vi "central core - noise.vi"() -> ()   [LabVIEW 2020]
uses:
  <vilib>/Analysis/3filter.llb/Filter Passband Type.ctl
  <vilib>/Utility/miscctls.llb/LVPointDoubleTypeDef.ctl
  <vilib>/Analysis/3filter.llb/Butterworth Filter (DBL).vi
  <vilib>/express/express analysis/Spectral/Block/exnSpectralBlock spectral measurements peak poly.vi
  <vilib>/express/express analysis/Spectral/Block/exnSpectralBlock spectral measurements peak WFM.vi
  <vilib>/express/express analysis/Spectral/XNode/ExpressSpectralMeasurementsBlockNode.xnode
  <vilib>/Analysis/NI_AALBase.lvlib
panel:
  out "Intensity Graph 3":dbl[][](graph)
  out "min value 2":dbl
  out "max value 2":dbl
  in  "low cutoff freq: fl":dbl=0.04 format="%#_13g"
  in  "order":i32=2
  in  "Array 3":cluster{dbl, "Color Box":u32}[](array[cluster])=[{1000.0, "Color Box"=16714752}, {750.0, "Color Box"=15859456}, {500.0, "Color Box"=65289}, {250.0, "Color Box"=983260}, {0.0, "Color Box"=14418124}]
  out "min value":dbl
  out "max value":dbl
  out "Array 2":dbl[][](array[numeric])
  out "Intensity Graph 2":dbl[][](graph)
  out "Waveform Graph 2":cluster{"f0":dbl, "df":dbl, "magnitude":dbl[]}(graph)
  out "Waveform Graph":cluster{"f0":dbl, "df":dbl, "magnitude":dbl[]}(graph)
  in  "Array":cluster{dbl, "Color Box":u32}[](array[cluster])=[{1000.0, "Color Box"=16714752}, {750.0, "Color Box"=15859456}, {500.0, "Color Box"=65289}, {250.0, "Color Box"=983260}, {0.0, "Color Box"=14418124}]
  out "output array":i16[](array[numeric])
  out "Image Pixels (I16) 2":i16[][](array[numeric])=[[45, 30, 48, 80, 127, 195, 237, 243, 154, 70, 122, 104, 194, 367, 352, 240, 149, 87, 63, 47, 92, 128, 128, 67, 39, 52, 45, 67, 104, 115], [50, 50, 64, 99, 81, 152, 118, 120, 92, 116, 64, 71, 100, 191, 192, 242, 150, 97, 76, 40, 47, 55, 45, 39, 54, 45, 64, 99, 149, 224], [37, 41, 43, 52, 61, 157, 144, 370, 413, 328, 136, 74, 77, 132, 154, 226, 274, 264, 263, 93, 47, 39, 36, 41, 45, 54, 64, 181, 262, 261], [57, 33, 48, 57, 36, 126, 400, 1139, 1471, 990, 426, 117, 68, 53, 213, 482, 730, 682, 502, 228, 70, 43, 50, 38, 46, 45, 63, 164, 233, 323], [42, 47, 36, 38, 50, 178, 708, 1307, 1980, 1298, 498, 186, 54, 79, 129, 508, 738, 836, 511, 332, 56, 51, 33, 48, 46, 47, 66, 133, 218, 251], [43, 33, 45, 58, 55, 122, 556, 966, 1092, 996, 478, 113, 88, 151, 232, 492, 730, 765, 572, 222, 84, 78, 52, 30, 29, 62, 43, 68, 94, 139], [49, 52, 36, 36, 42, 54, 167, 450, 516, 342, 265, 188, 394, 658, 854, 1048, 1097, 1085, 832, 485, 363, 136, 70, 48, 40, 27, 38, 48, 79, 82], [60, 41, 42, 40, 46, 44, 41, 105, 182, 261, 357, 707, 1036, 1348, 1662, 1687, 1948, 1605, 1319, 1576, 1082, 834, 344, 134, 50, 36, 42, 42, 48, 46], [36, 44, 51, 30, 51, 50, 58, 83, 234, 508, 950, 1428, 1764, 2324, 2186, 2166, 1882, 2127, 2020, 2238, 1880, 1490, 821, 427, 175, 65, 46, 45, 55, 56], [37, 42, 32, 33, 51, 44, 57, 161, 462, 1128, 1498, 1986, 2464, 2893, 2630, 2418, 2646, 3225, 3069, 2846, 2336, 1746, 1504, 1070, 494, 145, 72, 63, 36, 43], [50, 37, 40, 43, 41, 58, 120, 420, 986, 1616, 2419, 2510, 2533, 2588, 2872, 3422, 3455, 3263, 3008, 2527, 2411, 2560, 2122, 1861, 1150, 286, 77, 53, 41, 53], [40, 55, 58, 58, 46, 83, 257, 714, 1634, 1980, 2313, 2530, 2628, 2636, 3318, 3418, 3324, 3034, 2596, 2848, 2808, 3001, 2491, 1980, 1384, 651, 237, 40, 34, 48], [44, 40, 44, 45, 50, 130, 486, 1128, 1949, 2100, 2610, 2510, 3384, 3673, 3467, 3123, 2938, 2866, 3213, 3121, 3392, 3152, 2452, 1939, 1721, 1198, 510, 79, 41, 48], [33, 41, 40, 49, 45, 192, 763, 1254, 2019, 2332, 3095, 3363, 3632, 3650, 3081, 2909, 2967, 3495, 3610, 3411, 3053, 2633, 2652, 2554, 2042, 1442, 466, 78, 47, 45], [40, 46, 38, 43, 53, 203, 765, 1322, 1856, 2833, 3374, 3241, 3166, 2623, 2860, 3043, 3433, 3752, 3424, 2841, 2804, 2808, 3333, 2706, 2266, 1405, 691, 209, 52, 56], [42, 35, 46, 48, 75, 238, 777, 1499, 2356, 3159, 3058, 3150, 2850, 2866, 3378, 3538, 3456, 2992, 2823, 3076, 2986, 3476, 3549, 2923, 2054, 1364, 838, 259, 56, 70], [36, 46, 37, 48, 69, 183, 1109, 1898, 2624, 3005, 3002, 2850, 3306, 3476, 3378, 3509, 3199, 2884, 3449, 3510, 3308, 3642, 3143, 2620, 2131, 1809, 860, 256, 47, 56], [42, 44, 43, 38, 84, 216, 821, 1625, 2029, 2406, 2878, 3224, 3503, 3374, 3210, 2938, 2980, 3197, 3439, 3390, 3404, 3034, 2714, 2623, 2344, 1635, 1008, 185, 48, 47], [40, 67, 59, 58, 48, 210, 704, 1509, 1735, 2306, 3292, 3575, 3479, 3134, 2673, 3230, 3674, 3662, 3280, 3200, 2832, 3156, 3285, 2921, 2536, 1602, 722, 182, 49, 51], [46, 142, 147, 151, 72, 138, 433, 1157, 1793, 2633, 3124, 2894, 2851, 2854, 3294, 3636, 3774, 3640, 2965, 3071, 3170, 3313, 3315, 2559, 1880, 1187, 624, 85, 70, 43], [124, 201, 271, 363, 90, 64, 313, 820, 1802, 2216, 2614, 2334, 2950, 3845, 3980, 3365, 3359, 3001, 2949, 3217, 3262, 3548, 2841, 1976, 1393, 866, 296, 48, 47, 52], [132, 260, 538, 366, 212, 52, 135, 503, 1232, 1586, 2206, 2650, 3290, 3425, 3241, 2896, 2798, 3116, 3736, 3408, 3253, 2753, 2403, 1853, 1067, 564, 192, 58, 57, 35], [125, 225, 463, 371, 191, 78, 59, 238, 521, 1406, 1790, 2423, 2876, 2804, 2840, 3005, 3432, 3702, 3552, 3440, 2800, 2220, 1832, 1311, 826, 289, 82, 69, 44, 45], [99, 206, 331, 285, 222, 128, 264, 351, 516, 764, 1412, 2020, 2044, 2224, 2589, 2906, 2986, 3320, 2702, 2370, 2126, 1960, 1561, 672, 281, 75, 56, 38, 42, 47], [50, 64, 148, 147, 104, 132, 417, 735, 510, 468, 668, 893, 1382, 1918, 2400, 2465, 2452, 2236, 2205, 1993, 1615, 1078, 648, 239, 96, 49, 47, 36, 41, 50], [48, 56, 43, 67, 60, 150, 351, 731, 616, 378, 186, 384, 752, 878, 1230, 1220, 1315, 1364, 1133, 1140, 840, 448, 162, 66, 40, 36, 57, 50, 40, 43], [53, 47, 48, 59, 32, 90, 196, 410, 484, 183, 91, 60, 212, 250, 340, 452, 628, 495, 450, 302, 173, 86, 63, 43, 45, 43, 40, 41, 40, 42], [38, 38, 42, 37, 44, 46, 78, 142, 149, 115, 70, 52, 59, 54, 66, 80, 97, 69, 72, 46, 59, 50, 44, 55, 51, 40, 34, 42, 45, 39], [47, 42, 37, 50, 50, 42, 59, 53, 81, 41, 36, 52, 44, 62, 53, 44, 40, 42, 42, 47, 38, 47, 38, 55, 39, 57, 48, 41, 45, 47], [48, 47, 40, 37, 40, 50, 42, 35, 38, 48, 37, 61, 42, 53, 31, 46, 35, 38, 45, 37, 38, 34, 40, 32, 50, 36, 40, 57, 42, 46]]
  out "Intensity Graph":i16[][](graph)
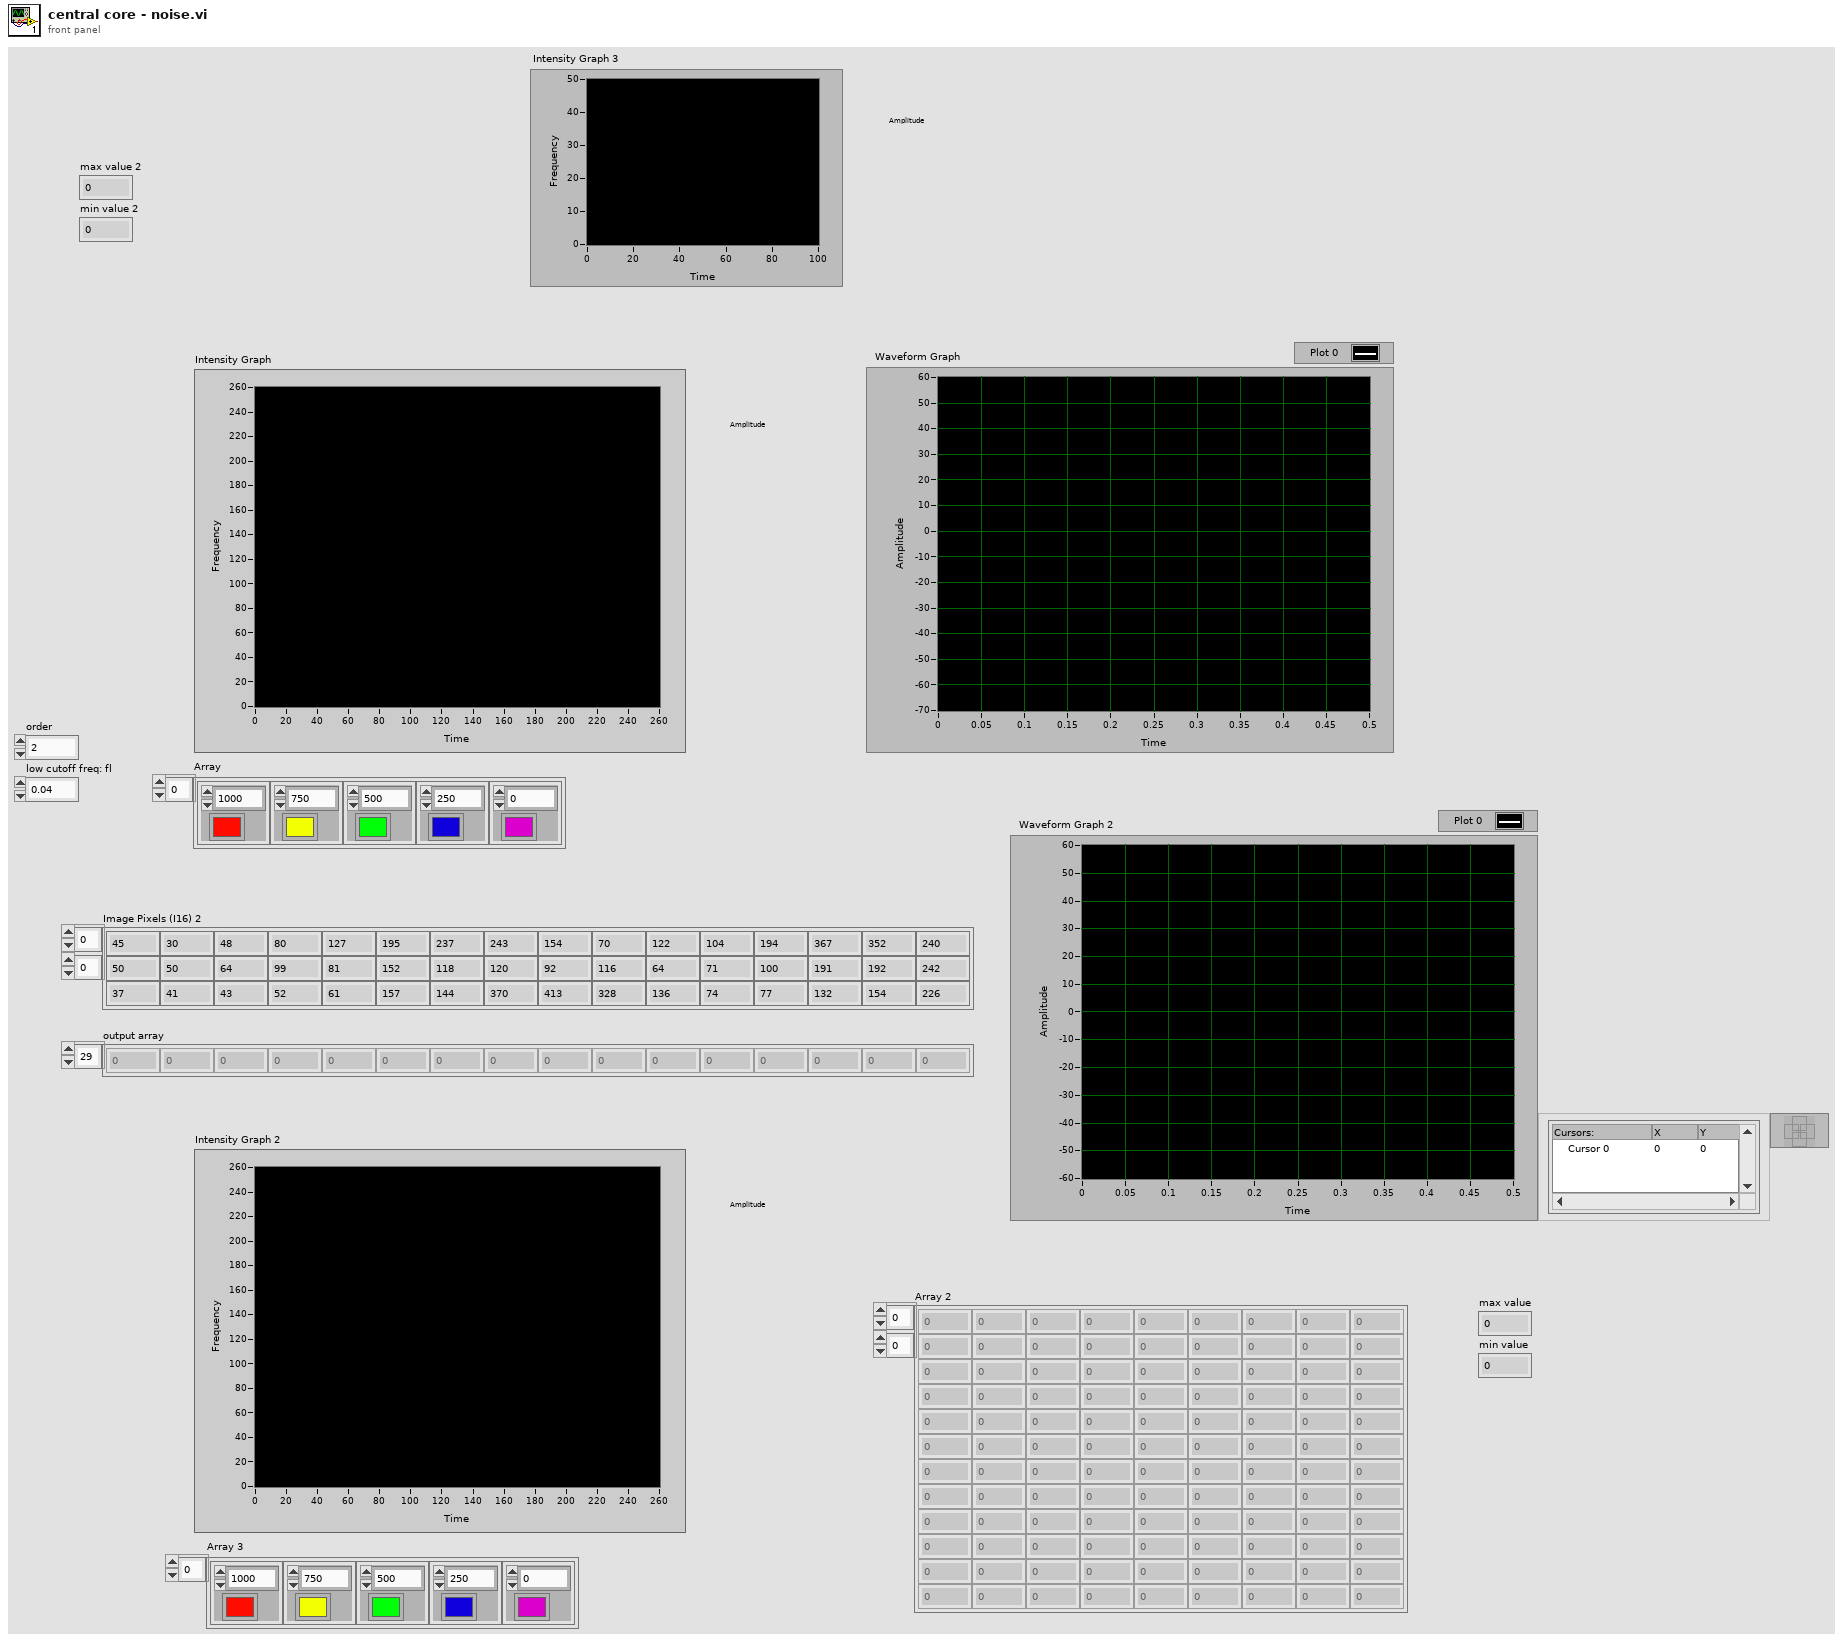
[diagram p1: front panel]
types:
  T1 = typedef "LVPointDoubleTypeDef.ctl" = cluster{"X":dbl, "Y":dbl}
  T2 = typedef "NI_AALBase.lvlib/Filter Passband Type.ctl" = enum32{"Lowpass", "Highpass", "Bandpass", "Bandstop"}
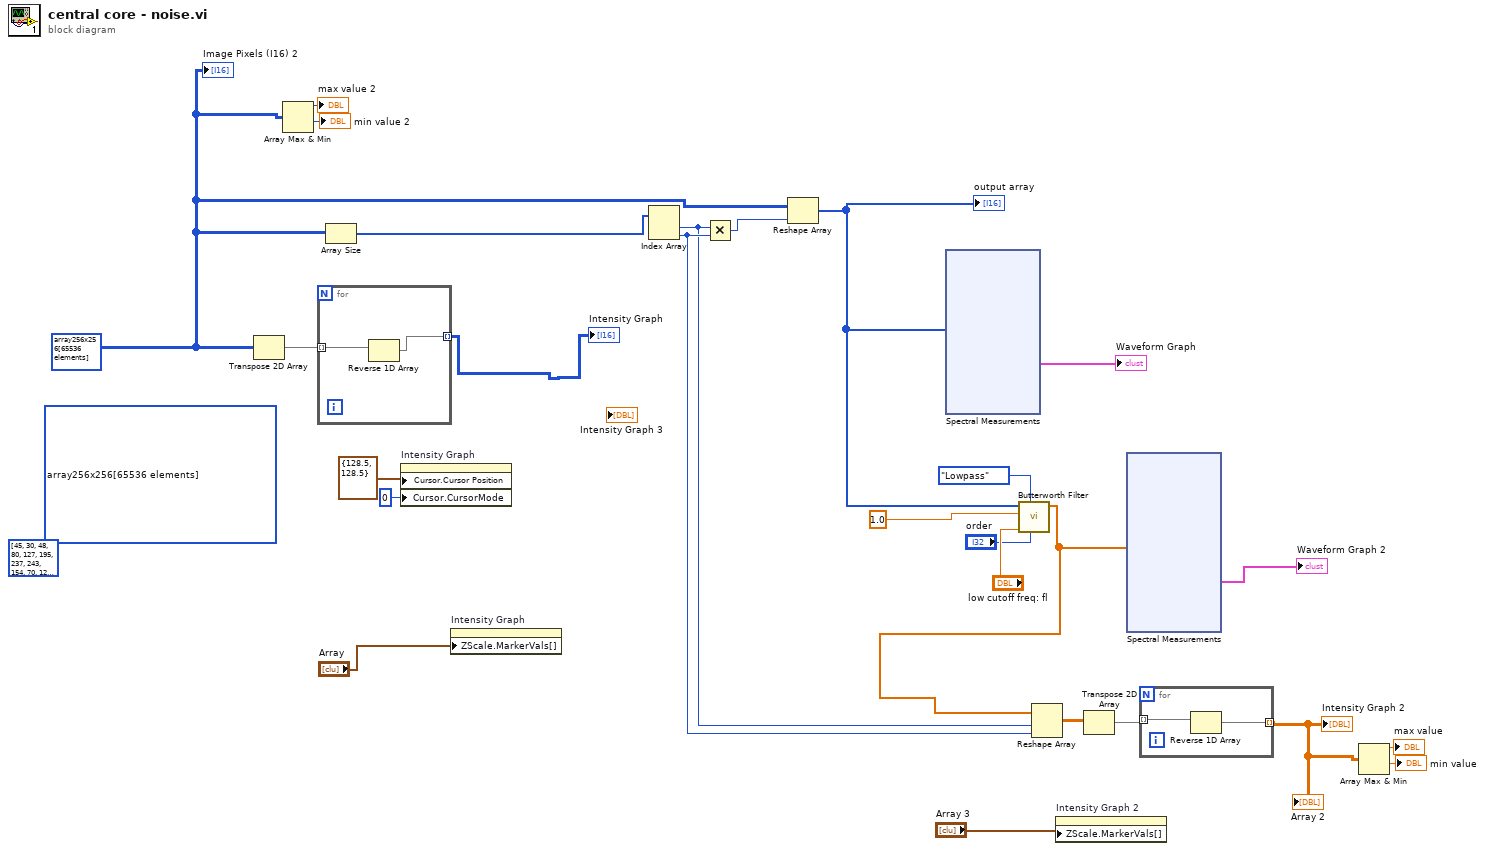
[diagram p0: block diagram]
diagram:
  (unwired) i16[][] array256x256[65536 elements] ("Image Pixels (I16)")
  w4 = i16[][] array256x256[65536 elements] ("Image Pixels (I16)")
  (unwired) i16[][] [[45, 30, 48, 80, 127, 195, 237, 243, 154, 70, 122, 104, 194, 367, 352, 240, 149, 87, 63, 47, 92, 128, 128, 67, 39, 52, 45, 67, 104, 115], [50, 50, 64, 99, 81, 152, 118, 120, 92, 116, 64, 71, 100, 191, 192, 242, 150, 97, 76, 40, 47, 55, 45, 39, 54, 45, 64, 99, 149, 224], [37, 41, 43, 52, 61, 157, 144, 370, 413, 328, 136, 74, 77, 132, 154, 226, 274, 264, 263, 93, 47, 39, 36, 41, 45, 54, 64, 181, 262, 261], [57, 33, 48, 57, 36, 126, 400, 1139, 1471, 990, 426, 117, 68, 53, 213, 482, 730, 682, 502, 228, 70, 43, 50, 38, 46, 45, 63, 164, 233, 323], [42, 47, 36, 38, 50, 178, 708, 1307, 1980, 1298, 498, 186, 54, 79, 129, 508, 738, 836, 511, 332, 56, 51, 33, 48, 46, 47, 66, 133, 218, 251], [43, 33, 45, 58, 55, 122, 556, 966, 1092, 996, 478, 113, 88, 151, 232, 492, 730, 765, 572, 222, 84, 78, 52, 30, 29, 62, 43, 68, 94, 139], [49, 52, 36, 36, 42, 54, 167, 450, 516, 342, 265, 188, 394, 658, 854, 1048, 1097, 1085, 832, 485, 363, 136, 70, 48, 40, 27, 38, 48, 79, 82], [60, 41, 42, 40, 46, 44, 41, 105, 182, 261, 357, 707, 1036, 1348, 1662, 1687, 1948, 1605, 1319, 1576, 1082, 834, 344, 134, 50, 36, 42, 42, 48, 46], [36, 44, 51, 30, 51, 50, 58, 83, 234, 508, 950, 1428, 1764, 2324, 2186, 2166, 1882, 2127, 2020, 2238, 1880, 1490, 821, 427, 175, 65, 46, 45, 55, 56], [37, 42, 32, 33, 51, 44, 57, 161, 462, 1128, 1498, 1986, 2464, 2893, 2630, 2418, 2646, 3225, 3069, 2846, 2336, 1746, 1504, 1070, 494, 145, 72, 63, 36, 43], [50, 37, 40, 43, 41, 58, 120, 420, 986, 1616, 2419, 2510, 2533, 2588, 2872, 3422, 3455, 3263, 3008, 2527, 2411, 2560, 2122, 1861, 1150, 286, 77, 53, 41, 53], [40, 55, 58, 58, 46, 83, 257, 714, 1634, 1980, 2313, 2530, 2628, 2636, 3318, 3418, 3324, 3034, 2596, 2848, 2808, 3001, 2491, 1980, 1384, 651, 237, 40, 34, 48], [44, 40, 44, 45, 50, 130, 486, 1128, 1949, 2100, 2610, 2510, 3384, 3673, 3467, 3123, 2938, 2866, 3213, 3121, 3392, 3152, 2452, 1939, 1721, 1198, 510, 79, 41, 48], [33, 41, 40, 49, 45, 192, 763, 1254, 2019, 2332, 3095, 3363, 3632, 3650, 3081, 2909, 2967, 3495, 3610, 3411, 3053, 2633, 2652, 2554, 2042, 1442, 466, 78, 47, 45], [40, 46, 38, 43, 53, 203, 765, 1322, 1856, 2833, 3374, 3241, 3166, 2623, 2860, 3043, 3433, 3752, 3424, 2841, 2804, 2808, 3333, 2706, 2266, 1405, 691, 209, 52, 56], [42, 35, 46, 48, 75, 238, 777, 1499, 2356, 3159, 3058, 3150, 2850, 2866, 3378, 3538, 3456, 2992, 2823, 3076, 2986, 3476, 3549, 2923, 2054, 1364, 838, 259, 56, 70], [36, 46, 37, 48, 69, 183, 1109, 1898, 2624, 3005, 3002, 2850, 3306, 3476, 3378, 3509, 3199, 2884, 3449, 3510, 3308, 3642, 3143, 2620, 2131, 1809, 860, 256, 47, 56], [42, 44, 43, 38, 84, 216, 821, 1625, 2029, 2406, 2878, 3224, 3503, 3374, 3210, 2938, 2980, 3197, 3439, 3390, 3404, 3034, 2714, 2623, 2344, 1635, 1008, 185, 48, 47], [40, 67, 59, 58, 48, 210, 704, 1509, 1735, 2306, 3292, 3575, 3479, 3134, 2673, 3230, 3674, 3662, 3280, 3200, 2832, 3156, 3285, 2921, 2536, 1602, 722, 182, 49, 51], [46, 142, 147, 151, 72, 138, 433, 1157, 1793, 2633, 3124, 2894, 2851, 2854, 3294, 3636, 3774, 3640, 2965, 3071, 3170, 3313, 3315, 2559, 1880, 1187, 624, 85, 70, 43], [124, 201, 271, 363, 90, 64, 313, 820, 1802, 2216, 2614, 2334, 2950, 3845, 3980, 3365, 3359, 3001, 2949, 3217, 3262, 3548, 2841, 1976, 1393, 866, 296, 48, 47, 52], [132, 260, 538, 366, 212, 52, 135, 503, 1232, 1586, 2206, 2650, 3290, 3425, 3241, 2896, 2798, 3116, 3736, 3408, 3253, 2753, 2403, 1853, 1067, 564, 192, 58, 57, 35], [125, 225, 463, 371, 191, 78, 59, 238, 521, 1406, 1790, 2423, 2876, 2804, 2840, 3005, 3432, 3702, 3552, 3440, 2800, 2220, 1832, 1311, 826, 289, 82, 69, 44, 45], [99, 206, 331, 285, 222, 128, 264, 351, 516, 764, 1412, 2020, 2044, 2224, 2589, 2906, 2986, 3320, 2702, 2370, 2126, 1960, 1561, 672, 281, 75, 56, 38, 42, 47], [50, 64, 148, 147, 104, 132, 417, 735, 510, 468, 668, 893, 1382, 1918, 2400, 2465, 2452, 2236, 2205, 1993, 1615, 1078, 648, 239, 96, 49, 47, 36, 41, 50], [48, 56, 43, 67, 60, 150, 351, 731, 616, 378, 186, 384, 752, 878, 1230, 1220, 1315, 1364, 1133, 1140, 840, 448, 162, 66, 40, 36, 57, 50, 40, 43], [53, 47, 48, 59, 32, 90, 196, 410, 484, 183, 91, 60, 212, 250, 340, 452, 628, 495, 450, 302, 173, 86, 63, 43, 45, 43, 40, 41, 40, 42], [38, 38, 42, 37, 44, 46, 78, 142, 149, 115, 70, 52, 59, 54, 66, 80, 97, 69, 72, 46, 59, 50, 44, 55, 51, 40, 34, 42, 45, 39], [47, 42, 37, 50, 50, 42, 59, 53, 81, 41, 36, 52, 44, 62, 53, 44, 40, 42, 42, 47, 38, 47, 38, 55, 39, 57, 48, 41, 45, 47], [48, 47, 40, 37, 40, 50, 42, 35, 38, 48, 37, 61, 42, 53, 31, 46, 35, 38, 45, 37, 38, 34, 40, 32, 50, 36, 40, 57, 42, 46]] ("Image Pixels (I16) 2")
  n1 = Transpose 2D Array(2D array=w4) -> (transposed array=w26:i16[][])
  n2 = Array Max & Min(array=w4) -> (max value=→"max value 2":i16, min value=→"min value 2":i16)  [unwired: 2 out]
  n3 = for {
    tunnel: w26 -> [w28] mode=indexing
    tunnel: [w27] -> w3 mode=indexing
    n4 = Reverse 1D Array(array=w28) -> (reversed array=w27:i16[])
  }
  "Intensity Graph" <- w3
  n5 = Array Size(array=w4) -> (size(s)=w25:i32[])
  n6 = property on="Intensity Graph" class="IntGraph (strict)"("Cursor.Cursor Position"=T1 {"X"=128.5, "Y"=128.5}, "Cursor.CursorMode"=u32 0 ("Cursor.Cursor Mode")) -> ()  [unwired: 2 in, 2 out]
  n7 = property on="Intensity Graph" class="IntGraph (strict)"("ZScale.MarkerVals[]"="Array") -> ()  [unwired: 2 in, 2 out]
  n8 = Index Array(array=w25) -> (element #1=w17:i32, element #2=w18:i32)  [unwired: 2 in]
  n9 = Multiply(x=w17, y=w18) -> (x*y=w24:i32)
  n10 = Reshape Array(w4, w24) -> (w16:i16[])
  "output array" <- w16
  n11 = xnode "Spectral Measurements"("Signals"=w16) -> ("FFT - (Peak)"=→"Waveform Graph":cluster{"f0":dbl, "df":dbl, "magnitude":dbl[]})  [unwired: 1 in, 2 out]
  n12 = call-poly <vilib>:"Butterworth Filter.vi"("order"="order", "filter type"=Filter_Passband_Type."Lowpass", "low cutoff freq: fl"="low cutoff freq: fl", "sampling freq: fs"=1.0, "X"=w16) -> ("Filtered X"=w13:dbl[])  [unwired: 3 in, 1 out]
  n13 = Reshape Array(w13, w17, w18) -> (w15:dbl[][])
  n14 = property on="Intensity Graph 2" class="IntGraph (strict)"("ZScale.MarkerVals[]"="Array 3") -> ()  [unwired: 2 in, 2 out]
  n15 = Transpose 2D Array(2D array=w15) -> (transposed array=w14:dbl[][])
  n16 = xnode "Spectral Measurements"("Signals"=w13) -> ("FFT - (Peak)"=→"Waveform Graph 2":cluster{"f0":dbl, "df":dbl, "magnitude":dbl[]})  [unwired: 1 in, 2 out]
  n17 = for {
    tunnel: w14 -> [w30] mode=indexing
    tunnel: [w29] -> w12 mode=indexing
    n18 = Reverse 1D Array(array=w30) -> (reversed array=w29:dbl[])
  }
  "Intensity Graph 2" <- w12
  "Array 2" <- w12
  n19 = Array Max & Min(array=w12) -> (max value=→"max value":dbl, min value=→"min value":dbl)  [unwired: 2 out]
  "Image Pixels (I16) 2" <- w4
